vi "treeInit.vi"(8 "error in":errorcluster, 10 "Configuration Paths":refnum<vi>, 11 "Tree Refnum":refnum<vi>) -> (0 "error out":errorcluster, 1 "Config Cluster out":T1, 4 "Script name":string="Test Script")   [LabVIEW 2011]
uses:
  Config cluster.ctl
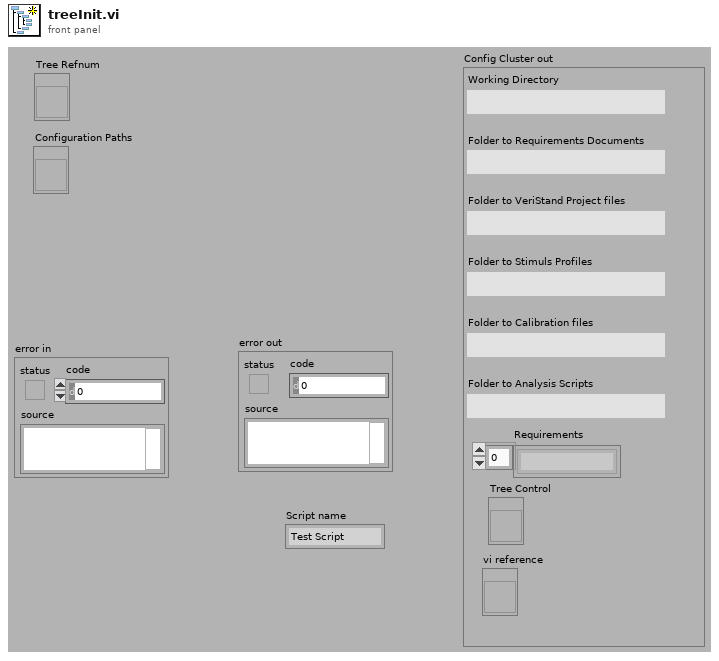
[diagram p1: front panel]
types:
  T1 = typedef "Config cluster.ctl" = cluster{"Working Directory":path, "Folder to Requirements Documents":path, "Folder to VeriStand Project files":path, "Folder to Stimuls Profiles":path, "Folder to Calibration files":path, "Folder to Analysis Scripts":path, "Requirements":string[], "Tree Control":refnum<vi>, "vi reference":refnum<vi>}
  T2 = typedef "imagedata.ctl" = cluster{"image type":i32, "image depth":i32, "image":u8[], "mask":u8[], "colors":u32[], "Rectangle":cluster{"left":i16, "top":i16, "right":i16, "bottom":i16}}
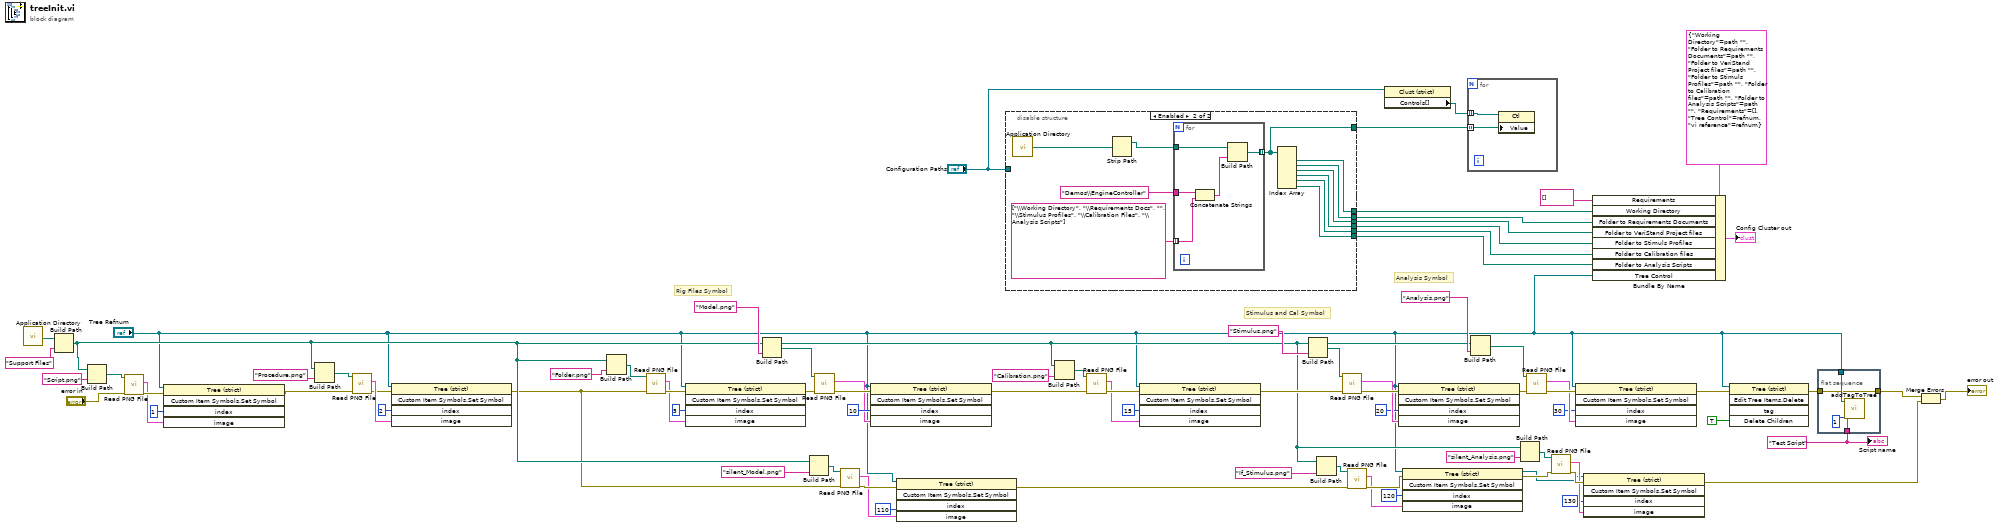
[diagram p0: block diagram]
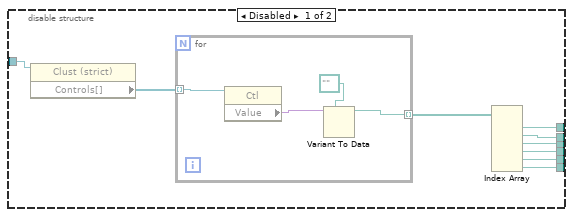
[diagram p2: hidden frame]
diagram:
  w51 = "Test Script" ("new tag")
  # "Analysis Symbol"
  # "Stimulus and Cal Symbol"
  # "Rig Files Symbol"
  n1 = call <vilib>:"Application Directory.vi"() -> ("Application Directory"=w4:path)
  n2 = Build Path(base path=w4, name or relative path="Support Files") -> (appended path=w14:path)
  n3 = Build Path(base path=w14, name or relative path="Script.png") -> (appended path=w44:path)
  n4 = call <vilib>:"Read PNG File.vi"("error in (no error)"="error in", "path to PNG file"=w44) -> ("error out"=w43:errorcluster, "image data"=w40:T2)  [unwired: 7 in, 1 out]
  n5 = invoke on="Invoke Node" class="Tree (strict)" method="Custom Item Symbols.Set Symbol"(reference="Tree Refnum", error in=w43, "index"=1 ("Index"), "image"=w40) -> (error out=w38:errorcluster)  [unwired: 1 in, 4 out]
  n6 = Build Path(base path=w14, name or relative path="Procedure.png") -> (appended path=w45:path)
  n7 = call <vilib>:"Read PNG File.vi"("error in (no error)"=w38, "path to PNG file"=w45) -> ("error out"=w46:errorcluster, "image data"=w48:T2)  [unwired: 7 in, 1 out]
  n8 = invoke on="Invoke Node" class="Tree (strict)" method="Custom Item Symbols.Set Symbol"(reference="Tree Refnum", error in=w46, "index"=2 ("Index"), "image"=w48) -> (error out=w7:errorcluster)  [unwired: 1 in, 4 out]
  n9 = Build Path(base path=w14, name or relative path="Folder.png") -> (appended path=w50:path)
  n10 = call <vilib>:"Read PNG File.vi"("error in (no error)"=w7, "path to PNG file"=w50) -> ("error out"=w65:errorcluster, "image data"=w62:T2)  [unwired: 7 in, 1 out]
  n11 = invoke on="Invoke Node" class="Tree (strict)" method="Custom Item Symbols.Set Symbol"(reference="Tree Refnum", error in=w65, "index"=5 ("Index"), "image"=w62) -> (error out=w64:errorcluster)  [unwired: 1 in, 4 out]
  n12 = Build Path(base path=w14, name or relative path="Model.png") -> (appended path=w71:path)
  n13 = Build Path(base path=w14, name or relative path="silent_Model.png") -> (appended path=w17:path)
  n14 = call <vilib>:"Read PNG File.vi"("error in (no error)"=w64, "path to PNG file"=w71) -> ("error out"=w79:errorcluster, "image data"=w73:T2)  [unwired: 7 in, 1 out]
  n15 = call <vilib>:"Read PNG File.vi"("error in (no error)"=w7, "path to PNG file"=w17) -> ("error out"=w15:errorcluster, "image data"=w13:T2)  [unwired: 7 in, 1 out]
  n16 = invoke on="Invoke Node" class="Tree (strict)" method="Custom Item Symbols.Set Symbol"(reference="Tree Refnum", error in=w79, "index"=10 ("Index"), "image"=w73) -> (error out=w36:errorcluster)  [unwired: 1 in, 4 out]
  n17 = invoke on="Invoke Node" class="Tree (strict)" method="Custom Item Symbols.Set Symbol"(reference="Tree Refnum", error in=w15, "index"=110 ("Index"), "image"=w13) -> (error out=w11:errorcluster)  [unwired: 1 in, 4 out]
  n18 = disable-structure shown="Enabled" {
    disable-tunnel: [w92 w103] -> w59
    disable-tunnel: [w91 w101] -> w58
    disable-tunnel: [w90 w100] -> w57
    disable-tunnel: [w89 w99] -> w56
    disable-tunnel: [w88 w98] -> w55
    disable-tunnel: [w87 w102] -> w53
    disable-tunnel: "Configuration Paths" -> [w86 _]
    disable-tunnel: [_ w97] -> w1
    frame Disabled {
      n19 = property class="Clust (strict)"(reference=w86) -> ("Controls[]"=w85:refnum<vi>[])  [unwired: 1 in, 2 out]
      n20 = for {
        tunnel: w85 -> [w96] mode=indexing
        tunnel: [w93] -> w84 mode=indexing
        n21 = property class="Ctl"(reference=w96) -> ("Value"=w95:variant)  [unwired: 1 in, 2 out]
        n22 = Variant To Data(type=path "", Variant=w95) -> (data=w93:path)  [unwired: 1 in, 1 out]
      }
      n23 = Index Array(array=w84) -> (element #1=w92:path, element #2=w87:path, element #3=w91:path, element #4=w90:path, element #5=w89:path, element #6=w88:path)  [unwired: 6 in]
    }
    frame Enabled {
      n24 = call <vilib>:"Application Directory.vi"() -> ("Application Directory"=w107:path)
      n25 = Strip Path(path=w107) -> (stripped path=w106:path)  [unwired: 1 out]
      n26 = for {
        tunnel: w106 -> [w112]
        tunnel: "Demos\\EngineController" -> [w111]
        tunnel: string[] ["\\Working Directory", "\\Requirements Docs", "", "\\Stimulus Profiles", "\\Calibration Files", "\\Analysis Scripts"] -> [w110] mode=indexing
        tunnel: [w108] -> w97 mode=indexing
        n27 = Concatenate Strings(w111, w110) -> (w109:string)
        n28 = Build Path(base path=w112, name or relative path=w109) -> (appended path=w108:path)
      }
      n29 = Index Array(array=w97) -> (element #1=w103:path, element #2=w102:path, element #3=w101:path, element #4=w100:path, element #5=w99:path, element #6=w98:path)  [unwired: 6 in]
    }
  }
  n30 = Build Path(base path=w14, name or relative path="Calibration.png") -> (appended path=w35:path)
  n31 = call <vilib>:"Read PNG File.vi"("error in (no error)"=w36, "path to PNG file"=w35) -> ("error out"=w34:errorcluster, "image data"=w31:T2)  [unwired: 7 in, 1 out]
  n32 = invoke on="Invoke Node" class="Tree (strict)" method="Custom Item Symbols.Set Symbol"(reference="Tree Refnum", error in=w34, "index"=15 ("Index"), "image"=w31) -> (error out=w33:errorcluster)  [unwired: 1 in, 4 out]
  n33 = Build Path(base path=w14, name or relative path="Stimulus.png") -> (appended path=w69:path)
  n34 = Build Path(base path=w14, name or relative path="If_Stimulus.png") -> (appended path=w29:path)
  n35 = call <vilib>:"Read PNG File.vi"("error in (no error)"=w33, "path to PNG file"=w69) -> ("error out"=w80:errorcluster, "image data"=w78:T2)  [unwired: 7 in, 1 out]
  n36 = call <vilib>:"Read PNG File.vi"("error in (no error)"=w11, "path to PNG file"=w29) -> ("error out"=w28:errorcluster, "image data"=w26:T2)  [unwired: 7 in, 1 out]
  n37 = property class="Clust (strict)"(reference="Configuration Paths") -> ("Controls[]"=w3:refnum<vi>[])  [unwired: 1 in, 2 out]
  n38 = invoke on="Invoke Node" class="Tree (strict)" method="Custom Item Symbols.Set Symbol"(reference="Tree Refnum", error in=w80, "index"=20 ("Index"), "image"=w78) -> (error out=w81:errorcluster)  [unwired: 1 in, 4 out]
  n39 = invoke on="Invoke Node" class="Tree (strict)" method="Custom Item Symbols.Set Symbol"(reference="Tree Refnum", error in=w28, "index"=120 ("Index"), "image"=w26) -> (reference out=w6:refnum<vi>, error out=w21:errorcluster)  [unwired: 1 in, 3 out]
  n40 = for {
    tunnel: w3 -> [w114] mode=indexing
    tunnel: w1 -> [w113] mode=indexing
    n41 = property class="Ctl"(reference=w114, "Value"=w113) -> ()  [unwired: 1 in, 2 out]
  }
  n42 = Build Path(base path=w14, name or relative path="Analysis.png") -> (appended path=w67:path)
  n43 = Build Path(base path=w14, name or relative path="silent_Analysis.png") -> (appended path=w23:path)
  n44 = call <vilib>:"Read PNG File.vi"("error in (no error)"=w81, "path to PNG file"=w67) -> ("error out"=w82:errorcluster, "image data"=w77:T2)  [unwired: 7 in, 1 out]
  n45 = call <vilib>:"Read PNG File.vi"("error in (no error)"=w21, "path to PNG file"=w23) -> ("error out"=w22:errorcluster, "image data"=w19:T2)  [unwired: 7 in, 1 out]
  n46 = invoke on="Invoke Node" class="Tree (strict)" method="Custom Item Symbols.Set Symbol"(reference="Tree Refnum", error in=w82, "index"=30 ("Index"), "image"=w77) -> (error out=w25:errorcluster)  [unwired: 1 in, 4 out]
  n47 = invoke on="Invoke Node" class="Tree (strict)" method="Custom Item Symbols.Set Symbol"(reference=w6, error in=w22, "index"=130 ("Index"), "image"=w19) -> (error out=w9:errorcluster)  [unwired: 1 in, 4 out]
  n48 = Bundle By Name(cluster=T1 {"Working Directory"=path "", "Folder to Requirements Documents"=path "", "Folder to VeriStand Project files"=path "", "Folder to Stimuls Profiles"=path "", "Folder to Calibration files"=path "", "Folder to Analysis Scripts"=path "", "Requirements"=[], "Tree Control"=refnum, "vi reference"=refnum} ("Configuration Paths"), "Requirements"=string[] [], "Working Directory"=w59, "Folder to Requirements Documents"=w53, "Folder to VeriStand Project files"=w58, "Folder to Stimuls Profiles"=w57, "Folder to Calibration files"=w56, "Folder to Analysis Scripts"=w55, "Tree Control"="Tree Refnum") -> (→"Config Cluster out":T1)
  n49 = invoke on="Invoke Node" class="Tree (strict)" method="Edit Tree Items.Delete"(reference="Tree Refnum", error in=w25, "Delete Children"=TRUE ("Delete Children?")) -> (error out=w24:errorcluster)  [unwired: 2 in, 4 out]
  n50 = flat-sequence {
    tunnel: w51 -> [w117]
    tunnel: "Tree Refnum" -> [w116]
    tunnel: w24 -> [w115]
    tunnel: [w115] -> w10
    frame #0 {
      n51 = call "addTagToTree.vi"("Tree ref"=w116, "new tag"=w117, "Symbol"=1) -> ()  [unwired: 12 in, 1 out]
    }
  }
  n52 = Merge Errors(w10, w9) -> (→"error out":errorcluster)
  "Script name" <- w51
